vi "Pop Up.vi"(11 "Dev Actor in":refnum<class "Dev Actor.lvclass">) -> (3 "Dev Actor out":refnum<class "Dev Actor.lvclass">)   [LabVIEW 2021, in "Dev Actor.lvlib" / "Dev Actor.lvclass"]
uses:
  Dev Actor.lvclass
  src/Actor/Msgs/Create/Create Msg/Create Msg.lvclass
  <vilib>/numeric/Random Number (Range) U64.vi
  Dev Panel/Dev Panel.lvclass
  src/Actor/Actor/Actor.lvclass
  C:/git/jettl/temp/Dev Actor/Dev Actor/Dev Actor.lvclass
  C:/git/jettl/temp/Msgs/Pop Up/Pop Up/Pop Up.lvclass
  C:/git/jettl/src/Actor/Actor/Actor.lvclass
  C:/git/jettl/src/Actor/Msgs/Create/Create/Create.lvclass
  C:/git/jettl/src/Actor/Msgs/Last Ack/Last Ack/Last Ack.lvclass
  C:/git/jettl/src/Actor/Msgs/Merge Error/Merge Error/Merge Error.lvclass
  C:/git/jettl/src/Actor/Msgs/Override Error/Override Error/Override Error.lvclass
  C:/git/jettl/src/Actor/Msgs/Teardown/Teardown/Teardown.lvclass
  C:/git/jettl/src/Actor/Msgs/Create/Create Msg/Create Msg.lvclass
  C:/git/jettl/src/Actor/Msg/Msg.lvclass
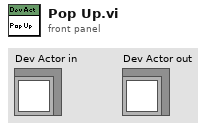
[diagram p1: front panel]
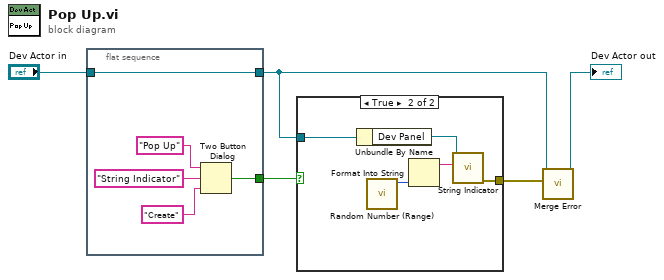
[diagram p0: block diagram]
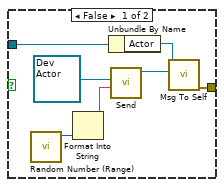
[diagram p2: hidden frame]
diagram:
  n1 = flat-sequence {
    tunnel: [w10] -> w1
    tunnel: "Dev Actor in" -> [w10]
    tunnel: [w7] -> w4
    frame #0 {
      n2 = Two Button Dialog(message="Pop Up", 1:"Create" ("F button name (\"Cancel\")"), 2:"String Indicator" ("T button name (\"OK\")")) -> (T button?=w7:bool)
    }
  }
  n3 = case shown="True" w4 {
    tunnel: w1 -> [w15 w22]
    tunnel: [w13 w18] -> w2
    frame False {
      n4 = call-poly <vilib>:"Random Number (Range).vi"() -> ("number"=w12:u64)  [unwired: 11 in]
      n5 = Format Into String(w12) -> (resulting string=w11:string)  [unwired: 3 in, 1 out]
      n6 = Unbundle By Name(w15) -> ("Actor"=w16:refnum<class "Actor.lvclass">)
      n7 = call "Send.vi"("Alias"=w11, "Actor"=refnum<class "Dev Actor.lvclass"> refnum ("Dev Actor.lvlib:Dev Actor.lvclass")) -> ("Create Msg out"=w14:refnum<class "Create Msg.lvclass">)  [unwired: 9 in]
      n8 = call-dynamic "Msg To Self.vi"("Msg"=w14, "Actor in"=w16) -> ("error out"=w13:errorcluster)  [unwired: 9 in]
    }
    frame True {
      n9 = Unbundle By Name(w22) -> ("Dev Panel"=w21:refnum<class "Dev Panel.lvclass">)
      n10 = call-poly <vilib>:"Random Number (Range).vi"() -> ("number"=w20:u64)  [unwired: 11 in]
      n11 = Format Into String(w20) -> (resulting string=w19:string)  [unwired: 3 in, 1 out]
      n12 = call "String Indicator.vi"("String Indicator"=w19, "Dev Panel in"=w21) -> ("error out"=w18:errorcluster)  [unwired: 9 in]
    }
  }
  n13 = call-dynamic "Merge Error.vi"("Error"=w2, "Dev Actor in"=w1) -> ("Dev Actor out"=→"Dev Actor out":refnum<class "Dev Actor.lvclass">)  [unwired: 9 in]
